vi "MALT Get One.vi"(8 "error in":errorcluster, 9 "port":i32, 10 "address":i32, 11 "cardType":i32) -> (0 "error out":errorcluster, 3 "status":bool)   [LabVIEW 2018]
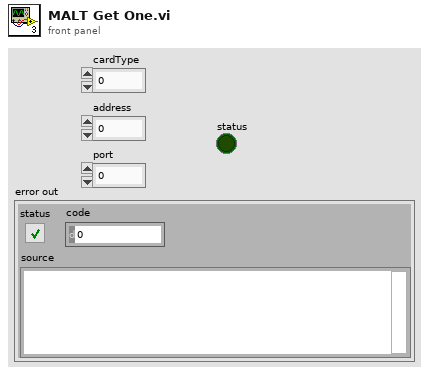
[diagram p1: front panel]
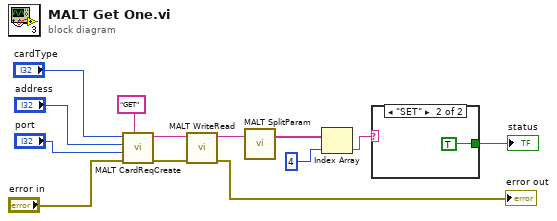
[diagram p0: block diagram]
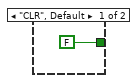
[diagram p2: hidden frame]
diagram:
  n1 = call "MALT CardReqCreate.vi"("cmd"="GET", "error in"="error in", "port"="port", "address"="address", "cardType"="cardType") -> ("error out"=w2:errorcluster, "request"=w7:string)  [unwired: 5 in]
  n2 = call "MALT WriteRead.vi"("error in"=w2, "data in"=w7) -> ("error out"=→"error out":errorcluster, "data out"=w13:string)  [unwired: 8 in]
  n3 = call "MALT SplitParam.vi"("line"=w13) -> ("items"=w11:string[])  [unwired: 2 in]
  n4 = Index Array(array=w11, index=4) -> (element=w9:string)
  n5 = case shown="\"SET\"" w9 {
    tunnel: [FALSE TRUE] -> w8
    frame "CLR", Default {
    }
    frame "SET" {
    }
  }
  "status" <- w8
